vi "Öffnen.vi"(8 "Error In":errorcluster caption="Fehler (Eingang)") -> (0 "Error Out":errorcluster caption="Fehler (Ausgang)", 3 "connection ID":refnum<k5>)   [LabVIEW 2024, in "Motor Treiber.lvlib"]
uses:
  Motor Treiber.lvlib
  SubVIs/Simulationsvariable.vi
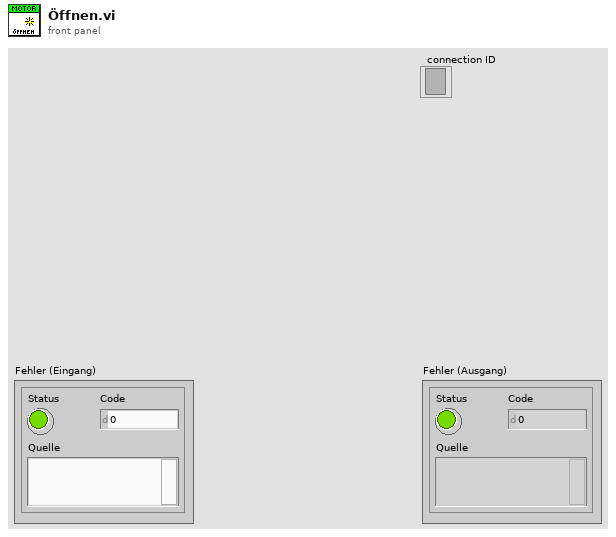
[diagram p1: front panel]
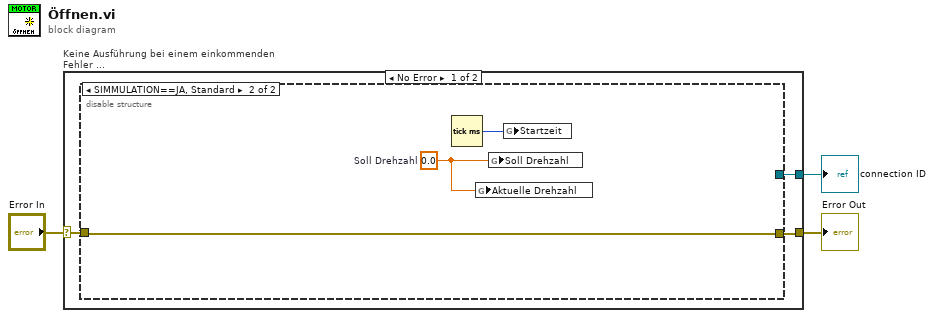
[diagram p0: block diagram]
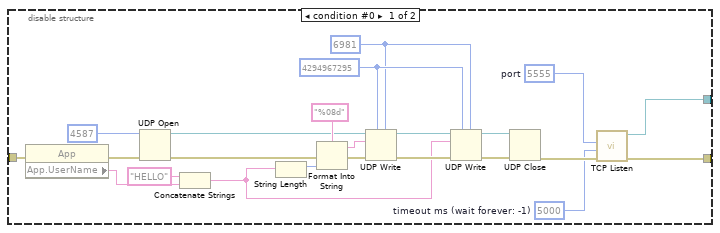
[diagram p2: hidden frame]
diagram:
  n1 = case "Keine Ausführung bei einem einkommenden Fehler ..." shown="No Error" "Error In" {
    selector: "Error In" -> [w6 w33]
    tunnel: [w4 w33] -> w2
    tunnel: [w5 _] -> w1
    frame No Error {
      n2 = disable-structure shown="SIMMULATION==JA, Standard" {
        disable-tunnel: w6 -> [w27 w32]
        disable-tunnel: [w22 _] -> w5
        disable-tunnel: [w21 w32] -> w4
        frame condition #0 {
          w7 = 5000  # timeout ms (wait forever: -1)
          w17 = u16 6981 ("Port oder Dienst")
          w18 = u32 4294967295 ("Adresse")
          w23 = u16 5555  # port
          n3 = property class="App"(error in=w27) -> (error out=w26:errorcluster, "App.UserName"=w25:string)  [unwired: 1 in, 1 out]
          n4 = UDP Open(8:w26, 11:u16 4587 ("Port")) -> (port=w10:refnum<k16>, 0:w12:errorcluster)  [unwired: 3 in, 1 out]
          n5 = Concatenate Strings("HELLO" ("Nachricht"), w25) -> (w11:string)
          n6 = String Length(string=w11) -> (length=w15:i32)
          n7 = Format Into String(format string="%08d" ("Format-String"), error in=w12, w15) -> (resulting string=w14:string, error out=w16:errorcluster)  [unwired: 1 in]
          n8 = UDP Write(address=w18, port or service name=w17, connection ID=w10, data in=w14, 8:w16) -> (error out=w20:errorcluster, 3:w19:refnum<k16>)  [unwired: 1 in]
          n9 = UDP Write(address=w18, port or service name=w17, connection ID=w19, data in=w11, 8:w20) -> (error out=w9:errorcluster, 3:w8:refnum<k16>)  [unwired: 1 in]
          n10 = UDP Close(connection ID=w8, 8:w9) -> (error out=w24:errorcluster)  [unwired: 1 out]
          n11 = call <vilib>:"TCP Listen.vi"("error in (no error)"=w24, "timeout ms (wait forever: -1)"=w7, "port"=w23) -> ("error out"=w21:errorcluster, "connection ID"=w22:refnum<k5>)  [unwired: 4 in, 3 out]
        }
        frame condition #1 (active) {
          w31 = 0.0  # Soll Drehzahl
          n12 = Tick Count (ms)() -> (millisecond timer value=w30:u32)
          n13 = global write "Simulationsvariable.vi" "Aktuelle Drehzahl"(w31) -> ()
          n14 = global write "Simulationsvariable.vi" "Soll Drehzahl"(w31) -> ()
          n15 = global write "Simulationsvariable.vi" "Startzeit"(w30) -> ()
        }
      }
    }
    frame Error {
    }
  }
  "Error Out" <- w2
  "connection ID" <- w1
